vi "带顺序排列组合.vi"(9 "组合i":i32[][](array[numeric]), 10 "不可等数值i":i32[](array[numeric]), 11 "数量":i32) -> (3 "组合o":i32[][](array[numeric]))   [LabVIEW 2017]
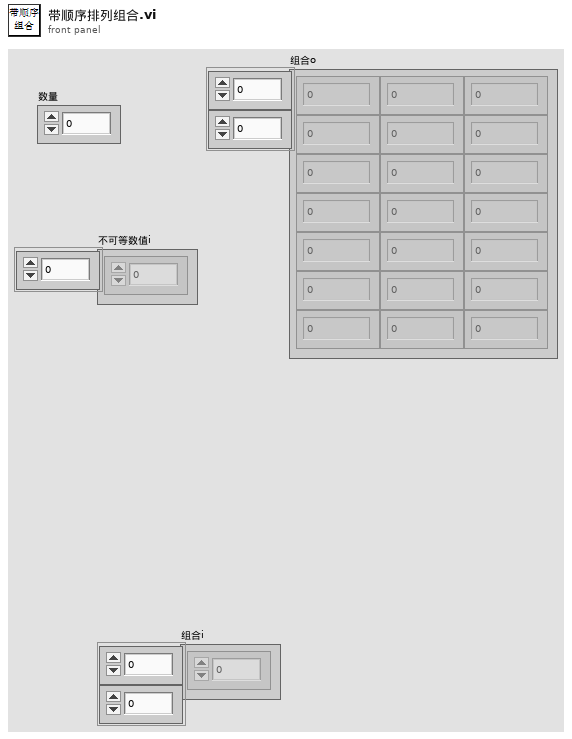
[diagram p1: front panel]
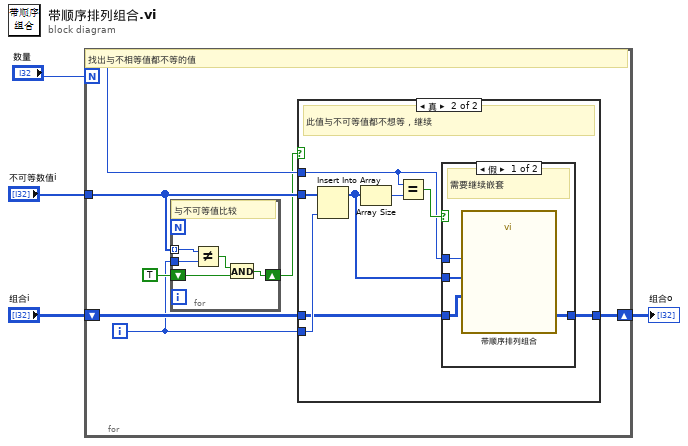
[diagram p0: block diagram]
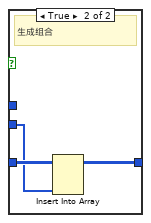
[diagram p3: hidden frame]
diagram:
  n1 = for {
    N: "数量" -> [w11]
    shift-right: [w10] -> w2
    shift-left: "组合i" -> [w9]
    tunnel: "不可等数值i" -> [w8]
    i -> [w5]
    # "找出与不相等值都不等的值"
    n2 = for {
      tunnel: w8 -> [w15] mode=indexing
      tunnel: w5 -> [w16]
      shift-right: [w14] -> w6
      shift-left: TRUE ("x != y?") -> [w13]
      # "与不可等值比较"
      n3 = Not Equal?(x=w15, y=w16) -> (x != y?=w12:bool)
      n4 = And(x=w12, y=w13) -> (x .and. y?=w14:bool)
    }
    n5 = case shown="真" w6 {
      tunnel: w8 -> [_ w19]
      tunnel: w11 -> [_ w20]
      tunnel: [w17 w21] -> w10
      tunnel: w9 -> [w17 w22]
      tunnel: w5 -> [_ w25]
      frame False {
        # "此值与不可等值中有相等，跳过"
      }
      frame True {
        # "此值与不可等值都不想等，继续"
        n6 = Insert Into Array(array=w19, new element=w25) -> (w18:i32[])  [unwired: 1 in]
        n7 = Array Size(array=w18) -> (size(s)=w24:i32)
        n8 = Equal?(x=w20, y=w24) -> (x = y?=w23:bool)
        n9 = case shown="假" w23 {
          tunnel: w20 -> [w29 _]
          tunnel: w22 -> [w28 w32]
          tunnel: [w27 w31] -> w21
          tunnel: w18 -> [w26 w30]
          frame False {
            # "需要继续嵌套"
            n10 = call "带顺序排列组合.vi"("组合i"=w28, "不可等数值i"=w26, "数量"=w29) -> ("组合o"=w27:i32[][])  [unwired: 8 in]
          }
          frame True {
            # "生成组合"
            n11 = Insert Into Array(array=w32, new element=w30) -> (w31:i32[][])  [unwired: 2 in]
          }
        }
      }
    }
  }
  "组合o" <- w2
